vi "Get Trigger Timer State.vi"(8 "error in (no error)":errorcluster, 10 "Timer (1)":i32=1 min=1 max=4 step=1 format="%#.6g", 11 "VISA resource name":refnum<visa-resource-name>) -> (0 "error out":errorcluster, 2 "Timer Enabled State":bool, 3 "VISA resource name out":refnum<visa-resource-name>)   [LabVIEW 2021, in "Keithley 2450.lvlib"]
doc: "This gets the status of the trigger timer."
uses:
  Keithley 2450.lvlib
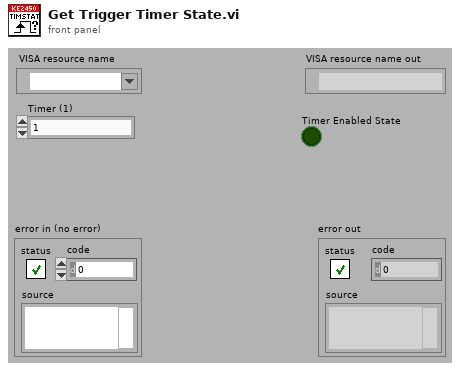
[diagram p1: front panel]
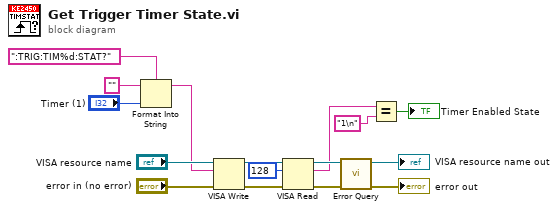
[diagram p0: block diagram]
diagram:
  n1 = Format Into String(format string=":TRIG:TIM%d:STAT?", initial string="", "Timer (1)") -> (resulting string=w9:string)  [unwired: 1 in, 1 out]
  n2 = VISA Write(VISA resource name="VISA resource name", write buffer=w9, error in (no error)="error in (no error)") -> (VISA resource name out=w6:refnum<visa-resource-name>, error out=w8:errorcluster)  [unwired: 1 out]
  n3 = VISA Read(VISA resource name=w6, byte count=u32 128, error in (no error)=w8) -> (VISA resource name out=w5:refnum<visa-resource-name>, read buffer=w1:string, error out=w7:errorcluster)  [unwired: 1 out]
  n4 = call "Error Query.vi"("error in (no error)"=w7, "VISA resource name"=w5) -> ("error out"=→"error out":errorcluster, "VISA resource name out"=→"VISA resource name out":refnum<visa-resource-name>)  [unwired: 8 out]
  n5 = Equal?(x=w1, y="1\n") -> (x = y?=→"Timer Enabled State":bool)
